vi "Initialise.vi"(8 "error in (no error)":errorcluster, 10 "Is Measuring Refnum":refnum<vi>, 11 "PalmSens in":refnum<class "PalmSens.lvclass">) -> (0 "error out":errorcluster, 3 "PalmSens out":refnum<class "PalmSens.lvclass">)   [LabVIEW 2025, in "PalmSens.lvclass"]
uses:
  PalmSens.lvclass
  PalmSens.lvclass/PalmSens.ctl
  E:/PSCode/PalmSens_SDK/labview/PalmSens/Libraries/PalmSens.Core.Simplified.LabVIEW.dll
  Libraries/PalmSens.Core.Simplified.LabVIEW.dll
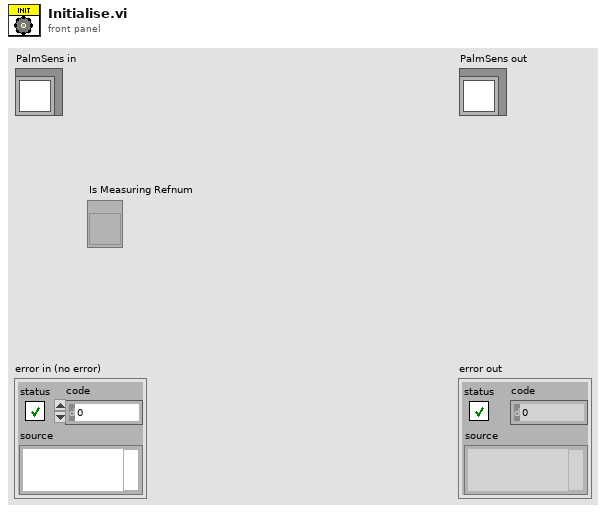
[diagram p1: front panel]
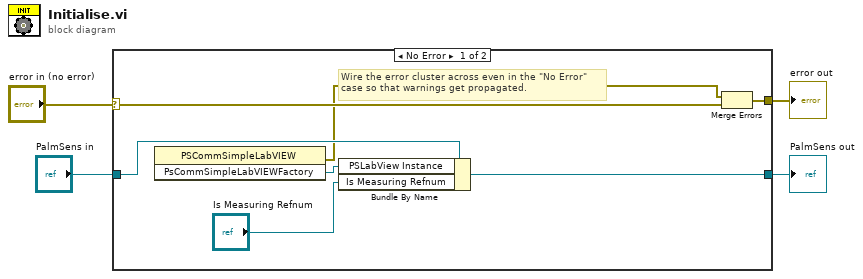
[diagram p0: block diagram]
diagram:
  n1 = case shown="No Error" "error in (no error)" {
    selector: "error in (no error)" -> [w11 w13]
    tunnel: [w10 w13] -> w3
    tunnel: [w8 w12] -> w1
    tunnel: "PalmSens in" -> [w9 w12]
    frame No Error {
      # "Wire the error cluster across even in the \"No Error\"\ncase so that warnings get propagated."
      n2 = invoke class="PSCommSimpleLabVIEW" method="PsCommSimpleLabVIEWFactory"() -> (error out=w5:errorcluster, "PsCommSimpleLabVIEWFactory"=w6:refnum<k24>)  [unwired: 3 in, 1 out]
      n3 = Bundle By Name(cluster=w9, "PSLabView Instance"=w6, "Is Measuring Refnum"="Is Measuring Refnum") -> (w8:refnum<class "PalmSens.lvclass">)
      n4 = Merge Errors(w5, w11) -> (w10:errorcluster)
    }
    frame Error {
    }
  }
  "error out" <- w3
  "PalmSens out" <- w1
